vi "Ballard - Arinc-429 Asynchronous RT Driver VI.vi"(10 "Parameters":variant, 11 "Process":refnum<class "Process.lvclass">) -> ()   [LabVIEW 2019, in "Ballard Arinc-429 Engine.lvlib"]
doc: "This VI is the Asynchronous VI for RT part."
uses:
  Ballard Arinc-429 Engine.lvlib
  <vilib>/NI/NIVS Inline Async API/_VS Inline Async API/Process/Process.lvclass
  <vilib>/NI/NIVS Inline Async API/_VS Inline Async API/Process/Process.lvclass/Process.ctl
  RT Controls/RT Asynchronous Parameters.ctl
  Shared/Controls and Global/RT HW Channel.ctl
  Shared/Controls and Global/RT Label Settings.ctl
  Shared/Controls and Global/Label.ctl
  Shared/Controls and Global/transferPeriod.ctl
  Shared/Controls and Global/RT Word Settings.ctl
  Shared/Controls and Global/RT Param Setting.ctl
  Shared/Controls and Global/Start Bit.ctl
  Shared/Controls and Global/Number of Bits.ctl
  <vilib>/NI VeriStand/Custom Device API/Block Data Reference.ctl
  <vilib>/NI VeriStand/Custom Device API/Data Reference.ctl
  <vilib>/NI VeriStand/Custom Device API/Custom Device Item Ref.ctl
  Shared/Controls and Global/TransferType.ctl
  RT Controls/Tx_Maps.ctl
  RT Controls/RT Tx Association.ctl
  RT Controls/RT Tx Default Raw Value.ctl
  RT Controls/RT Tx Default Raw Value_Association.ctl
  RT Controls/RT Tx Association Trigger Channels.ctl
  <vilib>/NI/NIVS Inline Async API/_Data Access Engine/Access Type Classes/ReadWrite/ReadWrite.lvclass/ReadWrite.ctl
  <vilib>/NI/NIVS Inline Async API/_Data Access Engine/Access Type Classes/Read/Read.lvclass/Read.ctl
  <vilib>/NI/NIVS Inline Async API/_Data Access Engine/Access Type Classes/Write/Write.lvclass/Write.ctl
  <vilib>/NI/NIVS Inline Async API/_Data Access Engine/Data Access Engine/Methods/Write.Data.vi
  <vilib>/NI/NIVS Inline Async API/_Data Access Engine/Data Access Engine/Methods/ReadWrite.Data.Reset.vi
  <vilib>/NI/NIVS Inline Async API/_Data Access Engine/Data Access Engine/Methods/Read.Data.vi
  <vilib>/NI/NIVS Inline Async API/_Data Access Engine/Data Access Engine/Methods/ReadWrite.Data.Read.vi
  <vilib>/NI/NIVS Inline Async API/_VS Inline Async API/Process/Data Member Access/Read Data Access.vi
  <vilib>/NI/NIVS Inline Async API/_VS Inline Async API/Error Handling Process/SubVIs/Error.ConvertArray.vi
  <vilib>/NI/NIVS Inline Async API/_Data Access Engine/Access Type Classes/Write/Write.ProcessData.vi
  <vilib>/NI/NIVS Inline Async API/_Data Access Engine/Access Type Classes/ReadWrite/ReadWrite.ProcessData.Reset.vi
  <vilib>/NI/NIVS Inline Async API/_Data Access Engine/Access Type Classes/Read/Read.ProcessData.vi
  <vilib>/NI/NIVS Inline Async API/_Data Access Engine/Access Type Classes/ReadWrite/ReadWrite.ProcessData.Read.vi
  <vilib>/NI/NIVS Inline Async API/_Data Access Engine/Data Access Engine/Methods/Read.Lookup.vi
  <vilib>/NI/NIVS Inline Async API/_Data Access Engine/Data Access Engine/Methods/ReadWrite.Lookup.vi
  <vilib>/NI/NIVS Inline Async API/_Data Access Engine/Data Access Engine/Methods/Write.Lookup.vi
  <vilib>/NI/NIVS Inline Async API/_Data Access Engine/Data Access Engine/Data Access Engine.lvclass
  Shared/Ballard Arinc-429 Shared.lvlib
  <vilib>/NI VeriStand/Custom Device API/Custom Device API.lvlib
panel:
  # "Custom Device Template\nv1.0"
  # "Use this template as a starting point for creating a custom device code module. The input controls shown here are specially named controls that the system will use to provide the device loop with data. The controls are not required for the device loop to run. For instance, if the device doesn't produce any output data, then you don't need the Device Outputs FIFO control. If you do use these controls, however, they need to have these exact names to be functional."
  # "The optional status notifier element is used to notify the RT engine of the last state of the custom device, and to indicate the device has completed execution. If this control is not used, a default No Error value is returned to the system when the device finishes execution.\n\nNote: This error state is not checked until the system shuts down. Use an output status channel to send more immediate status values to the system."
  # "This optional input can be used to send the VeriStand Engine the final status of the custom device initalization process. If this control exists on the custom device front panel, the VeriStand Engine will wait for a status update before starting up. If the custom device reports an error, that will abort the execution of the current configuration in the VeriStand Engine.\n\nThis control can be deleted if the custom device does not need to send the initialization status update."
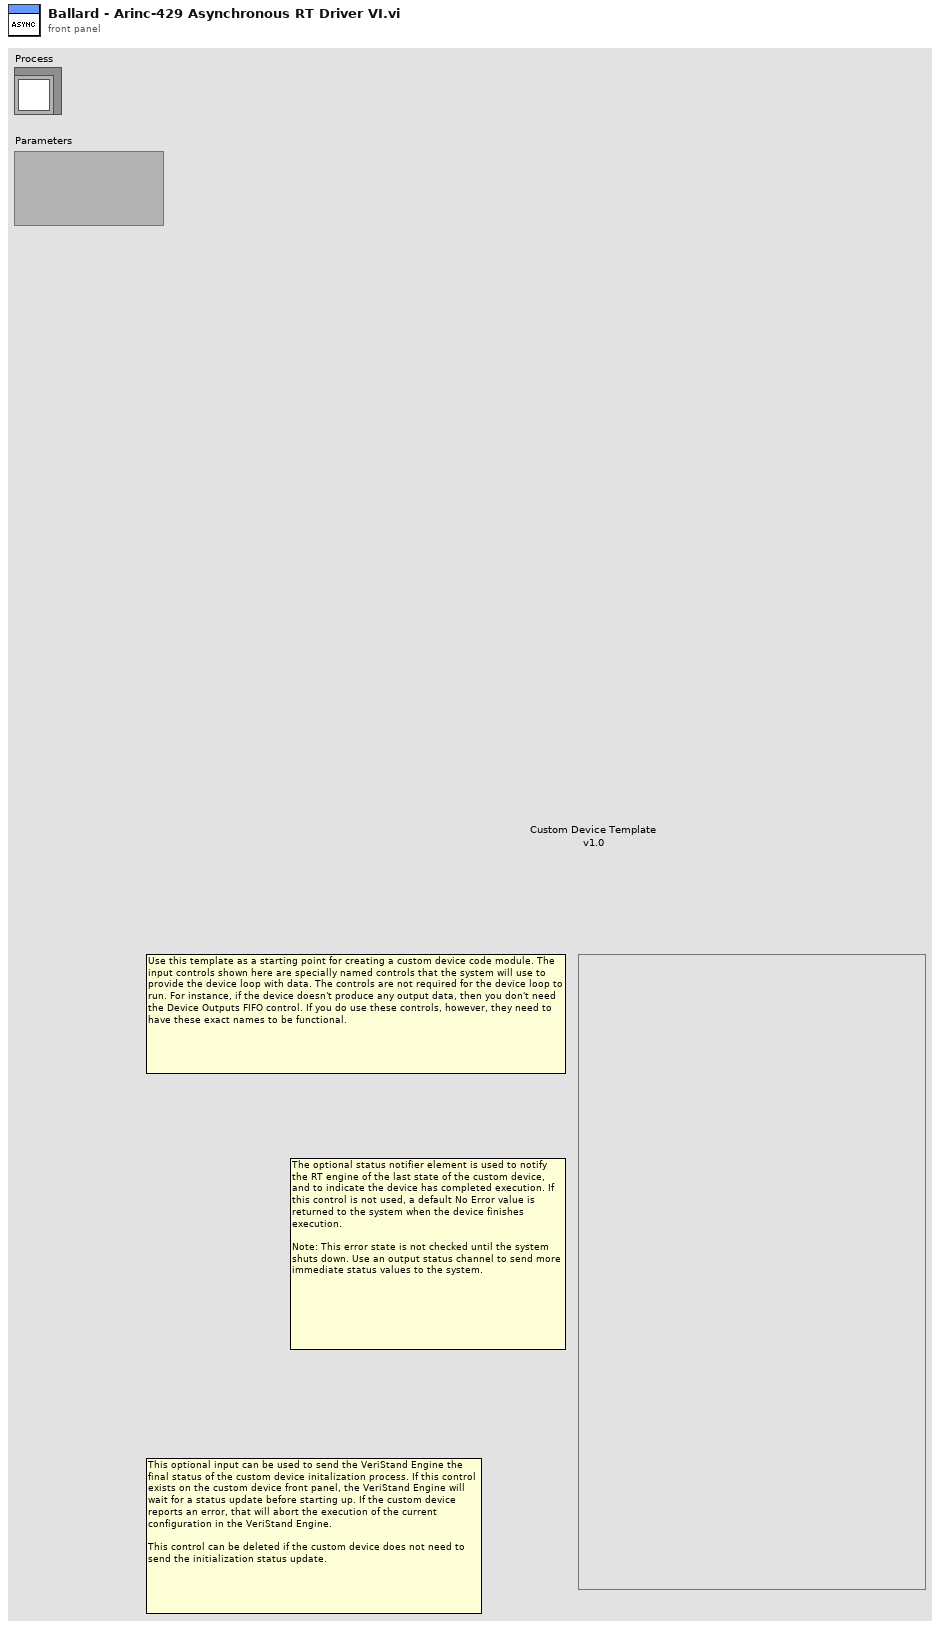
[diagram p1: front panel]
types:
  T1 = typedef "Ballard Arinc-429 Engine.lvlib/RT Asynchronous Parameters.ctl" = cluster{"Input Channel Data []":T2[], "Maps":T14, "core handle":u64}
  T2 = typedef "Ballard Arinc-429 Shared.lvlib/RT HW Channel.ctl" = cluster{"Labels Settings":T3[], "channel handle":u64, "channel #":u16}
  T3 = typedef "Ballard Arinc-429 Shared.lvlib/RT Label Settings.ctl" = cluster{"Name":string, "xmlName":string, "Label":T4, "transferPeriod":T5, "SDI_Enabled":bool, "SDI":u8, "Word":T6, "TransferType":T13, "has timestamp?":bool, "Label Disable/Trigger Channel Reference":T12, "Message Handle":u64, "Initialized?":bool, "Word Initial Raw Value":u32, "Label Timestamp Channel Data Reference":T11}
  T4 = typedef "Ballard Arinc-429 Shared.lvlib/Label.ctl" = u8
  T5 = typedef "Ballard Arinc-429 Shared.lvlib/transferPeriod.ctl" = u32
  T6 = typedef "Ballard Arinc-429 Shared.lvlib/RT Word Settings.ctl" = cluster{"Param Setting":T7}
  T7 = typedef "Ballard Arinc-429 Shared.lvlib/RT Param Setting.ctl" = cluster{"Start Bit":T8[], "Num Bits":T9[], "Signed?":bool[], "ScaleFac":dbl[], "ScaleOffset":dbl[], "Block Data Refs":T10[], "Encoding":enum16{"BNR", "BCD", "Discrete"}[], "Values Array":dbl[], "Item Refs":T12[]}
  T8 = typedef "Ballard Arinc-429 Shared.lvlib/Start Bit.ctl" = i32
  T9 = typedef "Ballard Arinc-429 Shared.lvlib/Number of Bits.ctl" = i32
  T10 = typedef "Custom Device API.lvlib/Block Data Reference.ctl" = cluster{"Data Reference":T11, "Offset":u64, "Length":u64}
  T11 = typedef "Custom Device API.lvlib/Data Reference.ctl" = i32
  T12 = typedef "Custom Device API.lvlib/Custom Device Item Ref.ctl" = u64
  T13 = typedef "Ballard Arinc-429 Shared.lvlib/TransferType.ctl" = enum16{"ScheduledLabel", "Acyclic", "Block", "Strobe"}
  T14 = typedef "Ballard Arinc-429 Engine.lvlib/Tx_Maps.ctl" = cluster{"Tx Map - Disable Channels":T15[], "Tx Map - Cyclic Labels - Parameters Channels":T15[], "Cyclic Labels - Raw Values":T16, "Tx Map - Trigger Channels":T18[], "Acyclic Labels - Raw Values":T16, "Tx Map - Acyclic Labels - Parameters Channels":T15[]}
  T15 = typedef "Ballard Arinc-429 Engine.lvlib/RT Tx Association.ctl" = cluster{"Channel Data Reference":T11, "Channel Index":i32, "Label Index":i32, "Parameter Index":i32, "Message Handle":u64, "Type":enum16{"Parameter Channel", "Disable/Trigger Channel"}}
  T16 = typedef "Ballard Arinc-429 Engine.lvlib/RT Tx Default Raw Value.ctl" = cluster{"Association":T17[], "Raw Values Array":u32[]}
  T17 = typedef "Ballard Arinc-429 Engine.lvlib/RT Tx Default Raw Value_Association.ctl" = cluster{"Channel Data Reference":T11, "Raw Value Index":i32}
  T18 = typedef "Ballard Arinc-429 Engine.lvlib/RT Tx Association Trigger Channels.ctl" = cluster{"Channel Data Reference":T11, "Channel Index":i32, "Label Index":i32, "Raw Value Index":i32, "channel handle":u64, "Type":enum16{"Parameter Channel", "Disable/Trigger Channel"}}
  T19 = typedef "Data Access Engine.lvlib/Data Access Engine.lvclass/Read.DVR.ctl" = refnum<data-value>
  T20 = typedef "Data Access Engine.lvlib/Data Access Engine.lvclass/ReadWrite.DVR.ctl" = refnum<data-value>
  T21 = typedef "Data Access Engine.lvlib/Data Access Engine.lvclass/Write.DVR.ctl" = refnum<data-value>
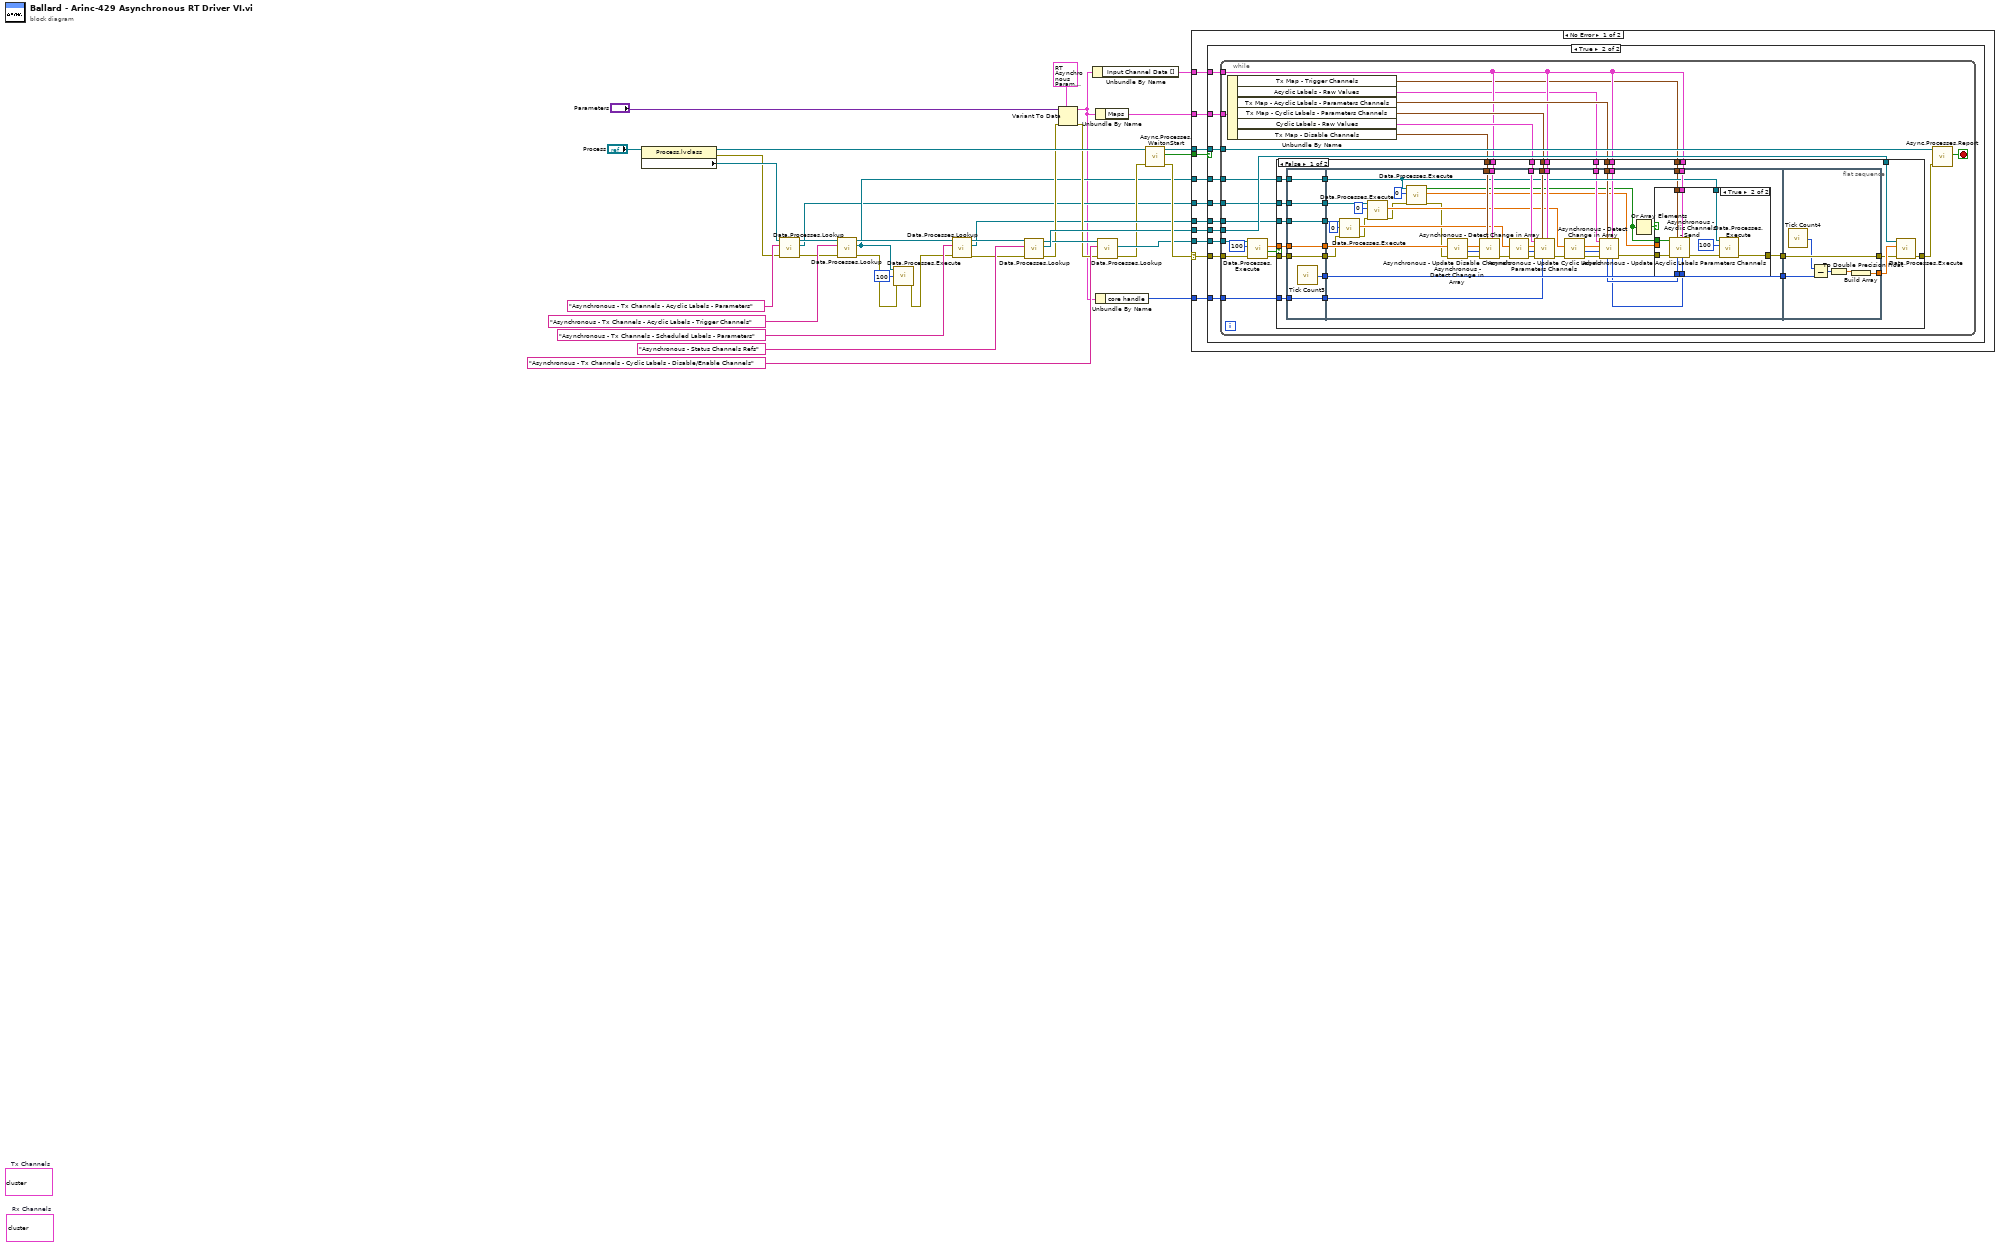
[diagram p0: block diagram]
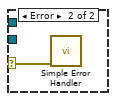
[diagram p5: hidden frame]
diagram:
  (unwired) T2[] [{"Labels Settings"=[{"Name"="label 1", "xmlName"="100", "Label"=23, "transferPeriod"=0, "SDI_Enabled"=FALSE, "SDI"=0, "Word"={"Param Setting"={"Start Bit"=[], "Num Bits"=[], "Signed?"=[], "ScaleFac"=[], "ScaleOffset"=[], "Block Data Refs"=[], "Encoding"=[], "Values Array"=[], "Item Refs"=[]}}, "TransferType"=enum."ScheduledLabel", "has timestamp?"=TRUE, "Label Disable/Trigger Channel Reference"=18446744073709551615, "Message Handle"=0, "Initialized?"=FALSE, "Word Initial Raw Value"=0, "Label Timestamp Channel Data Reference"=0}, {"Name"="label 2", "xmlName"="200", "Label"=24, "transferPeriod"=0, "SDI_Enabled"=FALSE, "SDI"=0, "Word"={"Param Setting"={"Start Bit"=[], "Num Bits"=[], "Signed?"=[], "ScaleFac"=[], "ScaleOffset"=[], "Block Data Refs"=[], "Encoding"=[], "Values Array"=[], "Item Refs"=[]}}, "TransferType"=enum."ScheduledLabel", "has timestamp?"=TRUE, "Label Disable/Trigger Channel Reference"=18446744073709551615, "Message Handle"=0, "Initialized?"=FALSE, "Word Initial Raw Value"=0, "Label Timestamp Channel Data Reference"=0}, {"Name"="label 3", "xmlName"="300", "Label"=25, "transferPeriod"=0, "SDI_Enabled"=FALSE, "SDI"=0, "Word"={"Param Setting"={"Start Bit"=[], "Num Bits"=[], "Signed?"=[], "ScaleFac"=[], "ScaleOffset"=[], "Block Data Refs"=[], "Encoding"=[], "Values Array"=[], "Item Refs"=[]}}, "TransferType"=enum."ScheduledLabel", "has timestamp?"=TRUE, "Label Disable/Trigger Channel Reference"=18446744073709551615, "Message Handle"=0, "Initialized?"=FALSE, "Word Initial Raw Value"=0, "Label Timestamp Channel Data Reference"=0}, {"Name"="label 4", "xmlName"="400", "Label"=26, "transferPeriod"=0, "SDI_Enabled"=FALSE, "SDI"=0, "Word"={"Param Setting"={"Start Bit"=[], "Num Bits"=[], "Signed?"=[], "ScaleFac"=[], "ScaleOffset"=[], "Block Data Refs"=[], "Encoding"=[], "Values Array"=[], "Item Refs"=[]}}, "TransferType"=enum."ScheduledLabel", "has timestamp?"=TRUE, "Label Disable/Trigger Channel Reference"=18446744073709551615, "Message Handle"=0, "Initialized?"=FALSE, "Word Initial Raw Value"=0, "Label Timestamp Channel Data Reference"=0}], "channel handle"=0, "channel #"=0}, {"Labels Settings"=[{"Name"="label 1", "xmlName"="101", "Label"=23, "transferPeriod"=0, "SDI_Enabled"=FALSE, "SDI"=0, "Word"={"Param Setting"={"Start Bit"=[], "Num Bits"=[], "Signed?"=[], "ScaleFac"=[], "ScaleOffset"=[], "Block Data Refs"=[], "Encoding"=[], "Values Array"=[], "Item Refs"=[]}}, "TransferType"=enum."ScheduledLabel", "has timestamp?"=TRUE, "Label Disable/Trigger Channel Reference"=18446744073709551615, "Message Handle"=0, "Initialized?"=FALSE, "Word Initial Raw Value"=0, "Label Timestamp Channel Data Reference"=0}, {"Name"="label 2", "xmlName"="201", "Label"=24, "transferPeriod"=0, "SDI_Enabled"=FALSE, "SDI"=0, "Word"={"Param Setting"={"Start Bit"=[], "Num Bits"=[], "Signed?"=[], "ScaleFac"=[], "ScaleOffset"=[], "Block Data Refs"=[], "Encoding"=[], "Values Array"=[], "Item Refs"=[]}}, "TransferType"=enum."ScheduledLabel", "has timestamp?"=TRUE, "Label Disable/Trigger Channel Reference"=18446744073709551615, "Message Handle"=0, "Initialized?"=FALSE, "Word Initial Raw Value"=0, "Label Timestamp Channel Data Reference"=0}, {"Name"="label 3", "xmlName"="301", "Label"=25, "transferPeriod"=0, "SDI_Enabled"=FALSE, "SDI"=0, "Word"={"Param Setting"={"Start Bit"=[], "Num Bits"=[], "Signed?"=[], "ScaleFac"=[], "ScaleOffset"=[], "Block Data Refs"=[], "Encoding"=[], "Values Array"=[], "Item Refs"=[]}}, "TransferType"=enum."ScheduledLabel", "has timestamp?"=TRUE, "Label Disable/Trigger Channel Reference"=18446744073709551615, "Message Handle"=0, "Initialized?"=FALSE, "Word Initial Raw Value"=0, "Label Timestamp Channel Data Reference"=0}, {"Name"="label 4", "xmlName"="401", "Label"=26, "transferPeriod"=0, "SDI_Enabled"=FALSE, "SDI"=0, "Word"={"Param Setting"={"Start Bit"=[], "Num Bits"=[], "Signed?"=[], "ScaleFac"=[], "ScaleOffset"=[], "Block Data Refs"=[], "Encoding"=[], "Values Array"=[], "Item Refs"=[]}}, "TransferType"=enum."ScheduledLabel", "has timestamp?"=TRUE, "Label Disable/Trigger Channel Reference"=18446744073709551615, "Message Handle"=0, "Initialized?"=FALSE, "Word Initial Raw Value"=0, "Label Timestamp Channel Data Reference"=0}, {"Name"="label 5", "xmlName"="501", "Label"=27, "transferPeriod"=0, "SDI_Enabled"=FALSE, "SDI"=0, "Word"={"Param Setting"={"Start Bit"=[], "Num Bits"=[], "Signed?"=[], "ScaleFac"=[], "ScaleOffset"=[], "Block Data Refs"=[], "Encoding"=[], "Values Array"=[], "Item Refs"=[]}}, "TransferType"=enum."ScheduledLabel", "has timestamp?"=TRUE, "Label Disable/Trigger Channel Reference"=18446744073709551615, "Message Handle"=0, "Initialized?"=FALSE, "Word Initial Raw Value"=0, "Label Timestamp Channel Data Reference"=0}, {"Name"="label 6", "xmlName"="601", "Label"=28, "transferPeriod"=0, "SDI_Enabled"=FALSE, "SDI"=0, "Word"={"Param Setting"={"Start Bit"=[], "Num Bits"=[], "Signed?"=[], "ScaleFac"=[], "ScaleOffset"=[], "Block Data Refs"=[], "Encoding"=[], "Values Array"=[], "Item Refs"=[]}}, "TransferType"=enum."ScheduledLabel", "has timestamp?"=TRUE, "Label Disable/Trigger Channel Reference"=18446744073709551615, "Message Handle"=0, "Initialized?"=FALSE, "Word Initial Raw Value"=0, "Label Timestamp Channel Data Reference"=0}], "channel handle"=0, "channel #"=1}, {"Labels Settings"=[{"Name"="label 1", "xmlName"="102", "Label"=23, "transferPeriod"=0, "SDI_Enabled"=FALSE, "SDI"=0, "Word"={"Param Setting"={"Start Bit"=[], "Num Bits"=[], "Signed?"=[], "ScaleFac"=[], "ScaleOffset"=[], "Block Data Refs"=[], "Encoding"=[], "Values Array"=[], "Item Refs"=[]}}, "TransferType"=enum."ScheduledLabel", "has timestamp?"=TRUE, "Label Disable/Trigger Channel Reference"=18446744073709551615, "Message Handle"=0, "Initialized?"=FALSE, "Word Initial Raw Value"=0, "Label Timestamp Channel Data Reference"=0}, {"Name"="label 2", "xmlName"="202", "Label"=24, "transferPeriod"=0, "SDI_Enabled"=FALSE, "SDI"=0, "Word"={"Param Setting"={"Start Bit"=[], "Num Bits"=[], "Signed?"=[], "ScaleFac"=[], "ScaleOffset"=[], "Block Data Refs"=[], "Encoding"=[], "Values Array"=[], "Item Refs"=[]}}, "TransferType"=enum."ScheduledLabel", "has timestamp?"=TRUE, "Label Disable/Trigger Channel Reference"=18446744073709551615, "Message Handle"=0, "Initialized?"=FALSE, "Word Initial Raw Value"=0, "Label Timestamp Channel Data Reference"=0}, {"Name"="label 3", "xmlName"="302", "Label"=25, "transferPeriod"=0, "SDI_Enabled"=FALSE, "SDI"=0, "Word"={"Param Setting"={"Start Bit"=[], "Num Bits"=[], "Signed?"=[], "ScaleFac"=[], "ScaleOffset"=[], "Block Data Refs"=[], "Encoding"=[], "Values Array"=[], "Item Refs"=[]}}, "TransferType"=enum."ScheduledLabel", "has timestamp?"=TRUE, "Label Disable/Trigger Channel Reference"=18446744073709551615, "Message Handle"=0, "Initialized?"=FALSE, "Word Initial Raw Value"=0, "Label Timestamp Channel Data Reference"=0}, {"Name"="label 4", "xmlName"="402", "Label"=26, "transferPeriod"=0, "SDI_Enabled"=FALSE, "SDI"=0, "Word"={"Param Setting"={"Start Bit"=[], "Num Bits"=[], "Signed?"=[], "ScaleFac"=[], "ScaleOffset"=[], "Block Data Refs"=[], "Encoding"=[], "Values Array"=[], "Item Refs"=[]}}, "TransferType"=enum."ScheduledLabel", "has timestamp?"=TRUE, "Label Disable/Trigger Channel Reference"=18446744073709551615, "Message Handle"=0, "Initialized?"=FALSE, "Word Initial Raw Value"=0, "Label Timestamp Channel Data Reference"=0}, {"Name"="label 5", "xmlName"="502", "Label"=27, "transferPeriod"=0, "SDI_Enabled"=FALSE, "SDI"=0, "Word"={"Param Setting"={"Start Bit"=[], "Num Bits"=[], "Signed?"=[], "ScaleFac"=[], "ScaleOffset"=[], "Block Data Refs"=[], "Encoding"=[], "Values Array"=[], "Item Refs"=[]}}, "TransferType"=enum."ScheduledLabel", "has timestamp?"=TRUE, "Label Disable/Trigger Channel Reference"=18446744073709551615, "Message Handle"=0, "Initialized?"=FALSE, "Word Initial Raw Value"=0, "Label Timestamp Channel Data Reference"=0}, {"Name"="label 6", "xmlName"="602", "Label"=28, "transferPeriod"=0, "SDI_Enabled"=FALSE, "SDI"=0, "Word"={"Param Setting"={"Start Bit"=[], "Num Bits"=[], "Signed?"=[], "ScaleFac"=[], "ScaleOffset"=[], "Block Data Refs"=[], "Encoding"=[], "Values Array"=[], "Item Refs"=[]}}, "TransferType"=enum."ScheduledLabel", "has timestamp?"=TRUE, "Label Disable/Trigger Channel Reference"=18446744073709551615, "Message Handle"=0, "Initialized?"=FALSE, "Word Initial Raw Value"=0, "Label Timestamp Channel Data Reference"=0}, {"Name"="label 7", "xmlName"="702", "Label"=29, "transferPeriod"=0, "SDI_Enabled"=FALSE, "SDI"=0, "Word"={"Param Setting"={"Start Bit"=[], "Num Bits"=[], "Signed?"=[], "ScaleFac"=[], "ScaleOffset"=[], "Block Data Refs"=[], "Encoding"=[], "Values Array"=[], "Item Refs"=[]}}, "TransferType"=enum."ScheduledLabel", "has timestamp?"=TRUE, "Label Disable/Trigger Channel Reference"=18446744073709551615, "Message Handle"=0, "Initialized?"=FALSE, "Word Initial Raw Value"=0, "Label Timestamp Channel Data Reference"=0}, {"Name"="label 8", "xmlName"="802", "Label"=30, "transferPeriod"=0, "SDI_Enabled"=FALSE, "SDI"=0, "Word"={"Param Setting"={"Start Bit"=[], "Num Bits"=[], "Signed?"=[], "ScaleFac"=[], "ScaleOffset"=[], "Block Data Refs"=[], "Encoding"=[], "Values Array"=[], "Item Refs"=[]}}, "TransferType"=enum."ScheduledLabel", "has timestamp?"=TRUE, "Label Disable/Trigger Channel Reference"=18446744073709551615, "Message Handle"=0, "Initialized?"=FALSE, "Word Initial Raw Value"=0, "Label Timestamp Channel Data Reference"=0}], "channel handle"=0, "channel #"=2}, {"Labels Settings"=[{"Name"="label 1 SDI 01", "xmlName"="10301", "Label"=23, "transferPeriod"=0, "SDI_Enabled"=FALSE, "SDI"=1, "Word"={"Param Setting"={"Start Bit"=[], "Num Bits"=[], "Signed?"=[], "ScaleFac"=[], "ScaleOffset"=[], "Block Data Refs"=[], "Encoding"=[], "Values Array"=[], "Item Refs"=[]}}, "TransferType"=enum."ScheduledLabel", "has timestamp?"=TRUE, "Label Disable/Trigger Channel Reference"=18446744073709551615, "Message Handle"=0, "Initialized?"=FALSE, "Word Initial Raw Value"=0, "Label Timestamp Channel Data Reference"=0}, {"Name"="label 1 SDI 11", "xmlName"="10311", "Label"=23, "transferPeriod"=0, "SDI_Enabled"=FALSE, "SDI"=3, "Word"={"Param Setting"={"Start Bit"=[], "Num Bits"=[], "Signed?"=[], "ScaleFac"=[], "ScaleOffset"=[], "Block Data Refs"=[], "Encoding"=[], "Values Array"=[], "Item Refs"=[]}}, "TransferType"=enum."ScheduledLabel", "has timestamp?"=TRUE, "Label Disable/Trigger Channel Reference"=18446744073709551615, "Message Handle"=0, "Initialized?"=FALSE, "Word Initial Raw Value"=0, "Label Timestamp Channel Data Reference"=0}, {"Name"="label 2", "xmlName"="203", "Label"=24, "transferPeriod"=0, "SDI_Enabled"=FALSE, "SDI"=0, "Word"={"Param Setting"={"Start Bit"=[], "Num Bits"=[], "Signed?"=[], "ScaleFac"=[], "ScaleOffset"=[], "Block Data Refs"=[], "Encoding"=[], "Values Array"=[], "Item Refs"=[]}}, "TransferType"=enum."ScheduledLabel", "has timestamp?"=TRUE, "Label Disable/Trigger Channel Reference"=18446744073709551615, "Message Handle"=0, "Initialized?"=FALSE, "Word Initial Raw Value"=0, "Label Timestamp Channel Data Reference"=0}], "channel handle"=0, "channel #"=3}]  # Rx Channels
  (unwired) T2[] [{"Labels Settings"=[{"Name"="label 1", "xmlName"="120", "Label"=23, "transferPeriod"=0, "SDI_Enabled"=FALSE, "SDI"=0, "Word"={"Param Setting"={"Start Bit"=[], "Num Bits"=[], "Signed?"=[], "ScaleFac"=[], "ScaleOffset"=[], "Block Data Refs"=[], "Encoding"=[], "Values Array"=[], "Item Refs"=[]}}, "TransferType"=enum."ScheduledLabel", "has timestamp?"=FALSE, "Label Disable/Trigger Channel Reference"=1, "Message Handle"=0, "Initialized?"=FALSE, "Word Initial Raw Value"=0, "Label Timestamp Channel Data Reference"=0}, {"Name"="label 2", "xmlName"="220", "Label"=24, "transferPeriod"=0, "SDI_Enabled"=FALSE, "SDI"=0, "Word"={"Param Setting"={"Start Bit"=[], "Num Bits"=[], "Signed?"=[], "ScaleFac"=[], "ScaleOffset"=[], "Block Data Refs"=[], "Encoding"=[], "Values Array"=[], "Item Refs"=[]}}, "TransferType"=enum."ScheduledLabel", "has timestamp?"=FALSE, "Label Disable/Trigger Channel Reference"=3, "Message Handle"=0, "Initialized?"=FALSE, "Word Initial Raw Value"=0, "Label Timestamp Channel Data Reference"=0}, {"Name"="label 3", "xmlName"="320", "Label"=25, "transferPeriod"=0, "SDI_Enabled"=FALSE, "SDI"=0, "Word"={"Param Setting"={"Start Bit"=[], "Num Bits"=[], "Signed?"=[], "ScaleFac"=[], "ScaleOffset"=[], "Block Data Refs"=[], "Encoding"=[], "Values Array"=[], "Item Refs"=[]}}, "TransferType"=enum."ScheduledLabel", "has timestamp?"=FALSE, "Label Disable/Trigger Channel Reference"=5, "Message Handle"=0, "Initialized?"=FALSE, "Word Initial Raw Value"=0, "Label Timestamp Channel Data Reference"=0}, {"Name"="label 4", "xmlName"="420", "Label"=26, "transferPeriod"=0, "SDI_Enabled"=FALSE, "SDI"=0, "Word"={"Param Setting"={"Start Bit"=[], "Num Bits"=[], "Signed?"=[], "ScaleFac"=[], "ScaleOffset"=[], "Block Data Refs"=[], "Encoding"=[], "Values Array"=[], "Item Refs"=[]}}, "TransferType"=enum."ScheduledLabel", "has timestamp?"=FALSE, "Label Disable/Trigger Channel Reference"=7, "Message Handle"=0, "Initialized?"=FALSE, "Word Initial Raw Value"=0, "Label Timestamp Channel Data Reference"=0}, {"Name"="label 5", "xmlName"="520", "Label"=27, "transferPeriod"=0, "SDI_Enabled"=FALSE, "SDI"=0, "Word"={"Param Setting"={"Start Bit"=[], "Num Bits"=[], "Signed?"=[], "ScaleFac"=[], "ScaleOffset"=[], "Block Data Refs"=[], "Encoding"=[], "Values Array"=[], "Item Refs"=[]}}, "TransferType"=enum."ScheduledLabel", "has timestamp?"=FALSE, "Label Disable/Trigger Channel Reference"=9, "Message Handle"=0, "Initialized?"=FALSE, "Word Initial Raw Value"=0, "Label Timestamp Channel Data Reference"=0}], "channel handle"=0, "channel #"=20}, {"Labels Settings"=[{"Name"="label 1", "xmlName"="121", "Label"=23, "transferPeriod"=0, "SDI_Enabled"=FALSE, "SDI"=0, "Word"={"Param Setting"={"Start Bit"=[], "Num Bits"=[], "Signed?"=[], "ScaleFac"=[], "ScaleOffset"=[], "Block Data Refs"=[], "Encoding"=[], "Values Array"=[], "Item Refs"=[]}}, "TransferType"=enum."ScheduledLabel", "has timestamp?"=FALSE, "Label Disable/Trigger Channel Reference"=11, "Message Handle"=0, "Initialized?"=FALSE, "Word Initial Raw Value"=0, "Label Timestamp Channel Data Reference"=0}, {"Name"="label 2", "xmlName"="221", "Label"=24, "transferPeriod"=0, "SDI_Enabled"=FALSE, "SDI"=0, "Word"={"Param Setting"={"Start Bit"=[], "Num Bits"=[], "Signed?"=[], "ScaleFac"=[], "ScaleOffset"=[], "Block Data Refs"=[], "Encoding"=[], "Values Array"=[], "Item Refs"=[]}}, "TransferType"=enum."ScheduledLabel", "has timestamp?"=FALSE, "Label Disable/Trigger Channel Reference"=13, "Message Handle"=0, "Initialized?"=FALSE, "Word Initial Raw Value"=0, "Label Timestamp Channel Data Reference"=0}, {"Name"="label 3", "xmlName"="321", "Label"=25, "transferPeriod"=0, "SDI_Enabled"=FALSE, "SDI"=0, "Word"={"Param Setting"={"Start Bit"=[], "Num Bits"=[], "Signed?"=[], "ScaleFac"=[], "ScaleOffset"=[], "Block Data Refs"=[], "Encoding"=[], "Values Array"=[], "Item Refs"=[]}}, "TransferType"=enum."ScheduledLabel", "has timestamp?"=FALSE, "Label Disable/Trigger Channel Reference"=15, "Message Handle"=0, "Initialized?"=FALSE, "Word Initial Raw Value"=0, "Label Timestamp Channel Data Reference"=0}, {"Name"="label 4", "xmlName"="421", "Label"=26, "transferPeriod"=0, "SDI_Enabled"=FALSE, "SDI"=0, "Word"={"Param Setting"={"Start Bit"=[], "Num Bits"=[], "Signed?"=[], "ScaleFac"=[], "ScaleOffset"=[], "Block Data Refs"=[], "Encoding"=[], "Values Array"=[], "Item Refs"=[]}}, "TransferType"=enum."ScheduledLabel", "has timestamp?"=FALSE, "Label Disable/Trigger Channel Reference"=17, "Message Handle"=0, "Initialized?"=FALSE, "Word Initial Raw Value"=0, "Label Timestamp Channel Data Reference"=0}, {"Name"="label 5", "xmlName"="521", "Label"=27, "transferPeriod"=0, "SDI_Enabled"=FALSE, "SDI"=0, "Word"={"Param Setting"={"Start Bit"=[], "Num Bits"=[], "Signed?"=[], "ScaleFac"=[], "ScaleOffset"=[], "Block Data Refs"=[], "Encoding"=[], "Values Array"=[], "Item Refs"=[]}}, "TransferType"=enum."ScheduledLabel", "has timestamp?"=FALSE, "Label Disable/Trigger Channel Reference"=19, "Message Handle"=0, "Initialized?"=FALSE, "Word Initial Raw Value"=0, "Label Timestamp Channel Data Reference"=0}, {"Name"="label 6", "xmlName"="621", "Label"=28, "transferPeriod"=0, "SDI_Enabled"=FALSE, "SDI"=0, "Word"={"Param Setting"={"Start Bit"=[], "Num Bits"=[], "Signed?"=[], "ScaleFac"=[], "ScaleOffset"=[], "Block Data Refs"=[], "Encoding"=[], "Values Array"=[], "Item Refs"=[]}}, "TransferType"=enum."ScheduledLabel", "has timestamp?"=FALSE, "Label Disable/Trigger Channel Reference"=21, "Message Handle"=0, "Initialized?"=FALSE, "Word Initial Raw Value"=0, "Label Timestamp Channel Data Reference"=0}, {"Name"="label 7", "xmlName"="721", "Label"=29, "transferPeriod"=0, "SDI_Enabled"=FALSE, "SDI"=0, "Word"={"Param Setting"={"Start Bit"=[], "Num Bits"=[], "Signed?"=[], "ScaleFac"=[], "ScaleOffset"=[], "Block Data Refs"=[], "Encoding"=[], "Values Array"=[], "Item Refs"=[]}}, "TransferType"=enum."ScheduledLabel", "has timestamp?"=FALSE, "Label Disable/Trigger Channel Reference"=23, "Message Handle"=0, "Initialized?"=FALSE, "Word Initial Raw Value"=0, "Label Timestamp Channel Data Reference"=0}], "channel handle"=0, "channel #"=21}, {"Labels Settings"=[{"Name"="label 1", "xmlName"="122", "Label"=23, "transferPeriod"=0, "SDI_Enabled"=FALSE, "SDI"=0, "Word"={"Param Setting"={"Start Bit"=[], "Num Bits"=[], "Signed?"=[], "ScaleFac"=[], "ScaleOffset"=[], "Block Data Refs"=[], "Encoding"=[], "Values Array"=[], "Item Refs"=[]}}, "TransferType"=enum."ScheduledLabel", "has timestamp?"=FALSE, "Label Disable/Trigger Channel Reference"=25, "Message Handle"=0, "Initialized?"=FALSE, "Word Initial Raw Value"=0, "Label Timestamp Channel Data Reference"=0}, {"Name"="label 2", "xmlName"="222", "Label"=24, "transferPeriod"=0, "SDI_Enabled"=FALSE, "SDI"=0, "Word"={"Param Setting"={"Start Bit"=[], "Num Bits"=[], "Signed?"=[], "ScaleFac"=[], "ScaleOffset"=[], "Block Data Refs"=[], "Encoding"=[], "Values Array"=[], "Item Refs"=[]}}, "TransferType"=enum."ScheduledLabel", "has timestamp?"=FALSE, "Label Disable/Trigger Channel Reference"=27, "Message Handle"=0, "Initialized?"=FALSE, "Word Initial Raw Value"=0, "Label Timestamp Channel Data Reference"=0}, {"Name"="label 3", "xmlName"="322", "Label"=25, "transferPeriod"=0, "SDI_Enabled"=FALSE, "SDI"=0, "Word"={"Param Setting"={"Start Bit"=[], "Num Bits"=[], "Signed?"=[], "ScaleFac"=[], "ScaleOffset"=[], "Block Data Refs"=[], "Encoding"=[], "Values Array"=[], "Item Refs"=[]}}, "TransferType"=enum."ScheduledLabel", "has timestamp?"=FALSE, "Label Disable/Trigger Channel Reference"=29, "Message Handle"=0, "Initialized?"=FALSE, "Word Initial Raw Value"=0, "Label Timestamp Channel Data Reference"=0}, {"Name"="label 4", "xmlName"="422", "Label"=26, "transferPeriod"=0, "SDI_Enabled"=FALSE, "SDI"=0, "Word"={"Param Setting"={"Start Bit"=[], "Num Bits"=[], "Signed?"=[], "ScaleFac"=[], "ScaleOffset"=[], "Block Data Refs"=[], "Encoding"=[], "Values Array"=[], "Item Refs"=[]}}, "TransferType"=enum."ScheduledLabel", "has timestamp?"=FALSE, "Label Disable/Trigger Channel Reference"=31, "Message Handle"=0, "Initialized?"=FALSE, "Word Initial Raw Value"=0, "Label Timestamp Channel Data Reference"=0}, {"Name"="label 5", "xmlName"="522", "Label"=27, "transferPeriod"=0, "SDI_Enabled"=FALSE, "SDI"=0, "Word"={"Param Setting"={"Start Bit"=[], "Num Bits"=[], "Signed?"=[], "ScaleFac"=[], "ScaleOffset"=[], "Block Data Refs"=[], "Encoding"=[], "Values Array"=[], "Item Refs"=[]}}, "TransferType"=enum."ScheduledLabel", "has timestamp?"=FALSE, "Label Disable/Trigger Channel Reference"=33, "Message Handle"=0, "Initialized?"=FALSE, "Word Initial Raw Value"=0, "Label Timestamp Channel Data Reference"=0}, {"Name"="label 6", "xmlName"="622", "Label"=28, "transferPeriod"=0, "SDI_Enabled"=FALSE, "SDI"=0, "Word"={"Param Setting"={"Start Bit"=[], "Num Bits"=[], "Signed?"=[], "ScaleFac"=[], "ScaleOffset"=[], "Block Data Refs"=[], "Encoding"=[], "Values Array"=[], "Item Refs"=[]}}, "TransferType"=enum."ScheduledLabel", "has timestamp?"=FALSE, "Label Disable/Trigger Channel Reference"=13, "Message Handle"=0, "Initialized?"=FALSE, "Word Initial Raw Value"=0, "Label Timestamp Channel Data Reference"=0}, {"Name"="label 7", "xmlName"="722", "Label"=29, "transferPeriod"=0, "SDI_Enabled"=FALSE, "SDI"=0, "Word"={"Param Setting"={"Start Bit"=[], "Num Bits"=[], "Signed?"=[], "ScaleFac"=[], "ScaleOffset"=[], "Block Data Refs"=[], "Encoding"=[], "Values Array"=[], "Item Refs"=[]}}, "TransferType"=enum."ScheduledLabel", "has timestamp?"=FALSE, "Label Disable/Trigger Channel Reference"=37, "Message Handle"=0, "Initialized?"=FALSE, "Word Initial Raw Value"=0, "Label Timestamp Channel Data Reference"=0}, {"Name"="label 8", "xmlName"="822", "Label"=30, "transferPeriod"=0, "SDI_Enabled"=FALSE, "SDI"=0, "Word"={"Param Setting"={"Start Bit"=[], "Num Bits"=[], "Signed?"=[], "ScaleFac"=[], "ScaleOffset"=[], "Block Data Refs"=[], "Encoding"=[], "Values Array"=[], "Item Refs"=[]}}, "TransferType"=enum."ScheduledLabel", "has timestamp?"=FALSE, "Label Disable/Trigger Channel Reference"=39, "Message Handle"=0, "Initialized?"=FALSE, "Word Initial Raw Value"=0, "Label Timestamp Channel Data Reference"=0}, {"Name"="label 9", "xmlName"="922", "Label"=31, "transferPeriod"=0, "SDI_Enabled"=FALSE, "SDI"=0, "Word"={"Param Setting"={"Start Bit"=[], "Num Bits"=[], "Signed?"=[], "ScaleFac"=[], "ScaleOffset"=[], "Block Data Refs"=[], "Encoding"=[], "Values Array"=[], "Item Refs"=[]}}, "TransferType"=enum."ScheduledLabel", "has timestamp?"=FALSE, "Label Disable/Trigger Channel Reference"=41, "Message Handle"=0, "Initialized?"=FALSE, "Word Initial Raw Value"=0, "Label Timestamp Channel Data Reference"=0}], "channel handle"=0, "channel #"=22}, {"Labels Settings"=[{"Name"="label 1", "xmlName"="123", "Label"=23, "transferPeriod"=0, "SDI_Enabled"=FALSE, "SDI"=0, "Word"={"Param Setting"={"Start Bit"=[], "Num Bits"=[], "Signed?"=[], "ScaleFac"=[], "ScaleOffset"=[], "Block Data Refs"=[], "Encoding"=[], "Values Array"=[], "Item Refs"=[]}}, "TransferType"=enum."ScheduledLabel", "has timestamp?"=FALSE, "Label Disable/Trigger Channel Reference"=43, "Message Handle"=0, "Initialized?"=FALSE, "Word Initial Raw Value"=0, "Label Timestamp Channel Data Reference"=0}], "channel handle"=0, "channel #"=23}]  # Tx Channels
  n1 = property class="Process.lvclass"(reference="Process") -> (reference out=w28:refnum<class "Process.lvclass">, error out=w9:errorcluster, "Data Member Access:Data Access"=w12:refnum<class "Data Access Engine.lvclass">)  [unwired: 1 in]
  n2 = call-poly <vilib>:"Data.Processes.Lookup.vi"("error in (no error)"=w9, "Name"="Asynchronous - Tx Channels - Acyclic Labels - Parameters", "Data Access API in"=w12) -> ("error out"=w10:errorcluster, "Ref"=w3:T19, "Data Access API out"=w11:refnum<class "Data Access Engine.lvclass">)  [unwired: 5 in, 1 out]
  n3 = call-poly <vilib>:"Data.Processes.Lookup.vi"("error in (no error)"=w10, "Name"="Asynchronous - Tx Channels - Acyclic Labels - Trigger Channels", "Data Access API in"=w11) -> ("error out"=w6:errorcluster, "Ref"=w7:T20, "Data Access API out"=w8:refnum<class "Data Access Engine.lvclass">)  [unwired: 5 in, 1 out]
  n4 = call-poly <vilib>:"Data.Processes.Execute.vi"("error in (no error)"=w6, "timeout ms"=100, "Ref"=w7) -> ("error out"=w5:errorcluster)  [unwired: 7 in, 1 out]
  n5 = call-poly <vilib>:"Data.Processes.Lookup.vi"("error in (no error)"=w5, "Name"="Asynchronous - Tx Channels - Scheduled Labels - Parameters", "Data Access API in"=w8) -> ("error out"=w18:errorcluster, "Ref"=w17:T19, "Data Access API out"=w19:refnum<class "Data Access Engine.lvclass">)  [unwired: 5 in, 1 out]
  n6 = call-poly <vilib>:"Data.Processes.Lookup.vi"("error in (no error)"=w18, "Name"="Asynchronous - Status Channels Refs", "Data Access API in"=w19) -> ("error out"=w23:errorcluster, "Ref"=w31:T21, "Data Access API out"=w30:refnum<class "Data Access Engine.lvclass">)  [unwired: 5 in, 1 out]
  n7 = Variant To Data(error in=w23, type=T1 {"Input Channel Data []"=[], "Maps"={"Tx Map - Disable Channels"=[], "Tx Map - Cyclic Labels - Parameters Channels"=[], "Cyclic Labels - Raw Values"={"Association"=[], "Raw Values Array"=[]}, "Tx Map - Trigger Channels"=[], "Acyclic Labels - Raw Values"={"Association"=[], "Raw Values Array"=[]}, "Tx Map - Acyclic Labels - Parameters Channels"=[]}, "core handle"=0} ("cluster"), Variant="Parameters") -> (data=w2:T1, error out=w22:errorcluster)
  n8 = Unbundle By Name(w2) -> ("Input Channel Data []"=w15:T2[])
  n9 = Unbundle By Name(w2) -> ("Maps"=w21:T14)
  n10 = Unbundle By Name(w2) -> ("core handle"=w1:u64)
  n11 = call-poly <vilib>:"Data.Processes.Lookup.vi"("error in (no error)"=w22, "Name"="Asynchronous - Tx Channels - Cyclic Labels - Disable/Enable Channels", "Data Access API in"=w30) -> ("error out"=w14:errorcluster, "Ref"=w32:T19)  [unwired: 5 in, 2 out]
  n12 = call <vilib>:"Async.Processes.WaitonStart.vi"("error in (no error)"=w14, "Process"=w28) -> ("error out"=w33:errorcluster, "Execute"=w35:bool, "Process out"=w34:refnum<class "Process.lvclass">)  [unwired: 7 in]
  n13 = case shown="No Error" w33 {
    selector: w33 -> [w42 w176]
    tunnel: w35 -> [w46 _]
    tunnel: w34 -> [w45 _]
    tunnel: w31 -> [w44 _]
    tunnel: w32 -> [w43 _]
    tunnel: w15 -> [w41 _]
    tunnel: w21 -> [w40 _]
    tunnel: w17 -> [w39 _]
    tunnel: w7 -> [w38 _]
    tunnel: w3 -> [w37 _]
    tunnel: w1 -> [w36 _]
    frame No Error {
      n14 = case shown="True" w46 {
        tunnel: w42 -> [_ w53]
        tunnel: w45 -> [_ w54]
        tunnel: w43 -> [_ w56]
        tunnel: w44 -> [_ w55]
        tunnel: w41 -> [_ w52]
        tunnel: w40 -> [_ w51]
        tunnel: w39 -> [_ w50]
        tunnel: w38 -> [_ w49]
        tunnel: w37 -> [_ w48]
        tunnel: w36 -> [_ w47]
        frame False {
        }
        frame True {
          n15 = while {
            tunnel: w53 -> [w74]
            tunnel: w54 -> [w78]
            tunnel: w56 -> [w76]
            tunnel: w55 -> [w75]
            tunnel: w52 -> [w61]
            tunnel: w51 -> [w70]
            tunnel: w50 -> [w68]
            tunnel: w49 -> [w64]
            tunnel: w48 -> [w63]
            tunnel: w47 -> [w57]
            stop <- w77 stop-if-true
            n16 = Unbundle By Name(w70) -> ("Tx Map - Trigger Channels"=w58:T18[], "Acyclic Labels - Raw Values"=w60:T16, "Tx Map - Acyclic Labels - Parameters Channels"=w62:T15[], "Tx Map - Cyclic Labels - Parameters Channels"=w66:T15[], "Cyclic Labels - Raw Values"=w65:T16, "Tx Map - Disable Channels"=w69:T15[])
            n17 = call-poly <vilib>:"Data.Processes.Execute.vi"("error in (no error)"=w74, "timeout ms"=100, "Ref"=w76) -> ("error out"=w71:errorcluster, "Timeout?"=w67:bool, "Values"=w72:dbl[])  [unwired: 6 in]
            n18 = case shown="False" w67 {
              tunnel: w75 -> [w101 _]
              tunnel: [w100 w175] -> w73
              tunnel: w72 -> [w99 _]
              tunnel: w71 -> [w98 w175]
              tunnel: w61 -> [w95 _]
              tunnel: w69 -> [w94 _]
              tunnel: w68 -> [w93 _]
              tunnel: w66 -> [w92 _]
              tunnel: w61 -> [w91 _]
              tunnel: w65 -> [w90 _]
              tunnel: w64 -> [w88 _]
              tunnel: w61 -> [w87 _]
              tunnel: w63 -> [w86 _]
              tunnel: w58 -> [w84 _]
              tunnel: w62 -> [w83 _]
              tunnel: w61 -> [w82 _]
              tunnel: w60 -> [w81 _]
              tunnel: w57 -> [w80 _]
              frame False {
                n19 = flat-sequence {
                  tunnel: w99 -> [w113]
                  tunnel: w98 -> [w114]
                  tunnel: [w114] -> w107
                  tunnel: [w113] -> w106
                  tunnel: [w112] -> w105
                  tunnel: w93 -> [w111]
                  tunnel: [w111] -> w104
                  tunnel: [w110] -> w89
                  tunnel: w88 -> [w110]
                  tunnel: w86 -> [w109]
                  tunnel: [w109] -> w85
                  tunnel: w80 -> [w108]
                  tunnel: [w108] -> w79
                  tunnel: w107 -> [w132]
                  tunnel: w106 -> [w156]
                  tunnel: [w146] -> w103
                  tunnel: w105 -> [w157]
                  tunnel: [w157] -> w102
                  tunnel: w95 -> [w155]
                  tunnel: w94 -> [w154]
                  tunnel: w104 -> [w153]
                  tunnel: w92 -> [w151]
                  tunnel: w91 -> [w150]
                  tunnel: w90 -> [w149]
                  tunnel: w89 -> [w147]
                  tunnel: w87 -> [w148]
                  tunnel: w85 -> [w145]
                  tunnel: w84 -> [w144]
                  tunnel: w83 -> [w139]
                  tunnel: w82 -> [w138]
                  tunnel: w81 -> [w137]
                  tunnel: w79 -> [w115]
                  tunnel: [w174] -> w96
                  tunnel: w103 -> [w174]
                  tunnel: w102 -> [w173]
                  tunnel: [w169] -> w97
                  frame #0 {
                    n20 = call "Tick Count3"() -> ("Tick Count(uSec)"=w112:u32)
                  }
                  frame #1 {
                    n21 = call-poly <vilib>:"Data.Processes.Execute.vi"("error in (no error)"=w132, "timeout ms"=0, "Ref"=w153) -> ("error out"=w119:errorcluster, "Values"=w152:dbl[])  [unwired: 6 in, 1 out]
                    n22 = call-poly <vilib>:"Data.Processes.Execute.vi"("error in (no error)"=w119, "timeout ms"=0, "Ref"=w145) -> ("error out"=w130:errorcluster, "Values"=w143:dbl[])  [unwired: 6 in, 1 out]
                    n23 = call-poly <vilib>:"Data.Processes.Execute.vi"("error in (no error)"=w130, "timeout ms"=0, "Ref"=w147) -> ("error out"=w129:errorcluster, "Data"=w134:dbl[], "Detect?"=w133:bool[])  [unwired: 5 in, 1 out]
                    n24 = call "Asynchronous - Detect Change in Array.vi"("Error (in)"=w129, "Data (in)"=w156) -> ("Error (out)"=w125:errorcluster, "Indexes"=w126:i32[], "Data (out)"=w127:dbl[])  [unwired: 7 in]
                    n25 = call "Asynchronous - Update Disable Channels.vi"("Channel Data []"=w155, "Map"=w154, "Error (in)"=w125, "Updated FIFO Index []"=w126, "Doubles []"=w127) -> ("Error (out)"=w121:errorcluster)  [unwired: 6 in]
                    n26 = call "Asynchronous - Detect Change in Array.vi"("Error (in)"=w121, "Data (in)"=w152) -> ("Error (out)"=w124:errorcluster, "Indexes"=w122:i32[], "Data (out)"=w123:dbl[])  [unwired: 7 in]
                    n27 = call "Asynchronous - Update Cyclic Labels Parameters Channels.vi"("Channel Data []"=w150, "core handle"=w115, "Map"=w151, "Error (in)"=w124, "Updated FIFO Index []"=w122, "Doubles []"=w123, "Raw Values"=w149) -> ("Error (out)"=w128:errorcluster)  [unwired: 4 in]
                    n28 = call "Asynchronous - Detect Change in Array.vi"("Error (in)"=w128, "Data (in)"=w143) -> ("Error (out)"=w142:errorcluster, "Indexes"=w141:i32[], "Data (out)"=w140:dbl[])  [unwired: 7 in]
                    n29 = call "Asynchronous - Update Acyclic Labels Parameters Channels.vi"("Channel Data []"=w138, "Map"=w139, "Error (in)"=w142, "Updated FIFO Index []"=w141, "Doubles []"=w140, "Raw Values"=w137) -> ("Error (out)"=w131:errorcluster, "Raw Values Array"=w135:u32[], "Raw Value Index"=w136:i32[])  [unwired: 3 in]
                    n30 = Or Array Elements(Boolean array=w133) -> (logical OR=w116:bool)
                    n31 = case shown="True" w116 {
                      tunnel: w131 -> [w158 w164]
                      tunnel: w148 -> [_ w168]
                      tunnel: w147 -> [_ w167]
                      tunnel: [w158 w165] -> w146
                      tunnel: w144 -> [_ w163]
                      tunnel: w136 -> [_ w162]
                      tunnel: w135 -> [_ w161]
                      tunnel: w134 -> [_ _]
                      tunnel: w133 -> [_ w159]
                      frame False {
                      }
                      frame True {
                        n32 = call "Asynchronous - Acyclic Channels - Send.vi"("Raw Values Array"=w161, "Channel Data []"=w168, "Raw Values Index Array"=w162, "Tx Map - Trigger Channels"=w163, "Error (in)"=w164, "Changes?"=w159) -> ("Error (out)"=w166:errorcluster)  [unwired: 5 in]
                        n33 = call-poly <vilib>:"Data.Processes.Execute.vi"("error in (no error)"=w166, "timeout ms"=100, "Ref"=w167) -> ("error out"=w165:errorcluster)  [unwired: 7 in, 1 out]
                      }
                    }
                  }
                  frame #2 {
                    n34 = call "Tick Count4"() -> ("Tick Count(uSec)"=w172:u32)
                    n35 = Subtract(x=w172, y=w173) -> (x-y=w171:u32)
                    n36 = To Double Precision Float(number=w171) -> (double precision float=w170:dbl)
                    n37 = Build Array(w170) -> (w169:dbl[])
                  }
                }
                n38 = call-poly <vilib>:"Data.Processes.Execute.vi"("error in (no error)"=w96, "Values"=w97, "Ref"=w101) -> ("error out"=w100:errorcluster)  [unwired: 8 in]
              }
              frame True {
              }
            }
            n39 = call <vilib>:"Async.Processes.Report.vi"("Error"=w73, "Process in"=w78) -> ("Stop"=w77:bool)  [unwired: 8 in, 1 out]
          }
        }
      }
    }
    frame Error {
      n40 = call <vilib>:"Simple Error Handler.vi"("error in (no error)"=w176) -> ()  [unwired: 4 in, 5 out]
    }
  }
